vi "PositionCalibration2.vi"() -> ()   [LabVIEW 2017]
uses:
  <vilib>/Analysis/baseanly.llb/Mean (DBL).vi
  <vilib>/Instr/_visa.llb/VISA Configure Serial Port (Instr).vi
  <vilib>/Analysis/NI_AALBase.lvlib
panel:
  out "Digitial Signal":dbl
  out "Read Buffer":string
  out "Write Buffer":string
  in  "Sample Rate (Hz)":dbl
  in  "Baud Rate":i32(ring) items=["9600"=9600, "115200"=115200]
  in  "COM Port":refnum<visa-resource-name>
  in  "Stop":bool
  in  "Start":bool
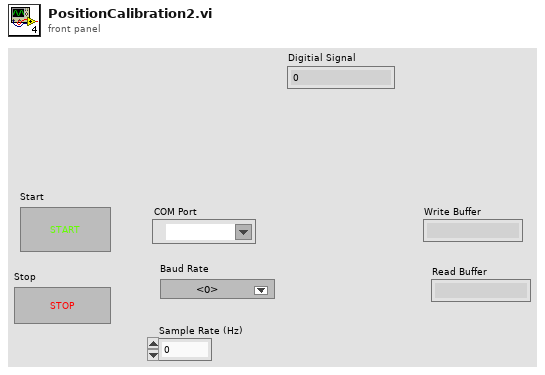
[diagram p1: front panel]
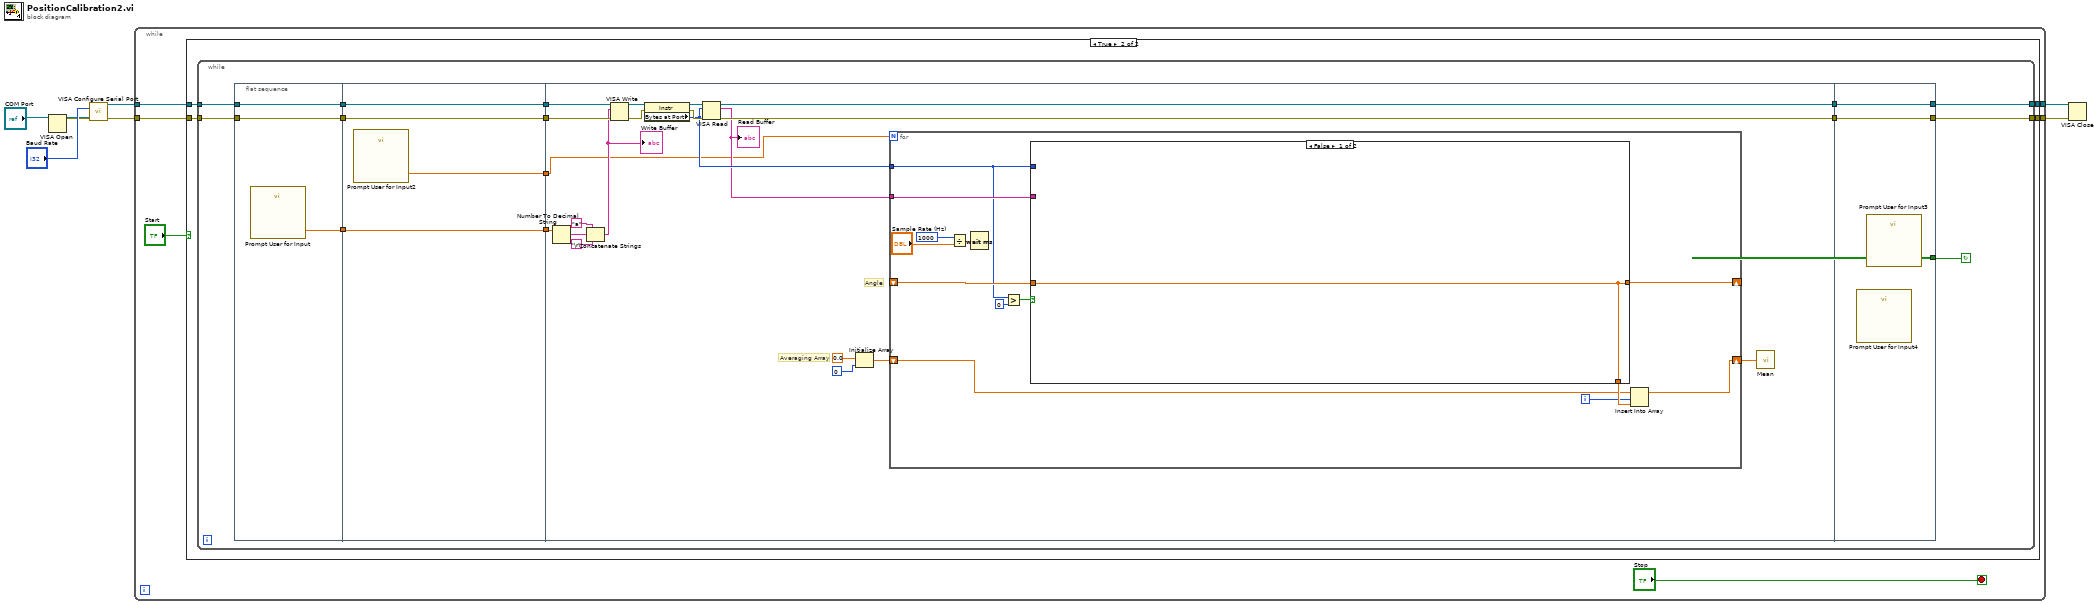
[diagram p0: block diagram]
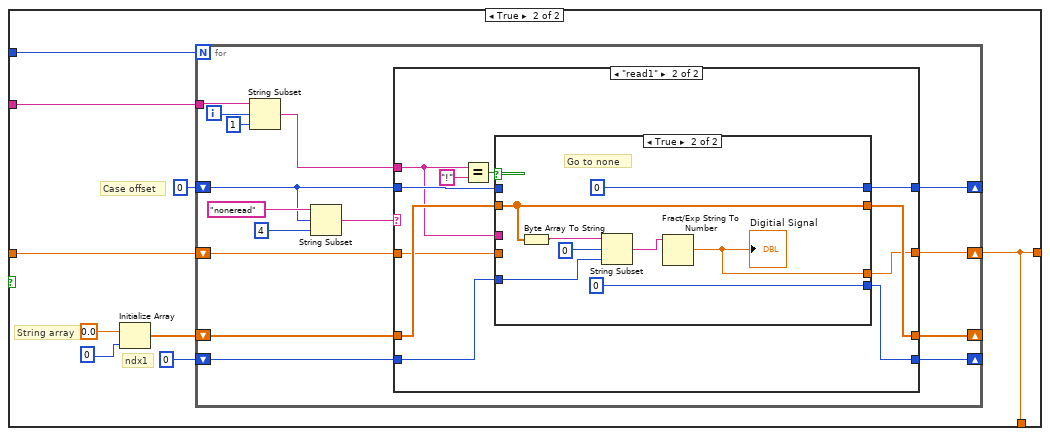
[diagram p3: hidden frame]
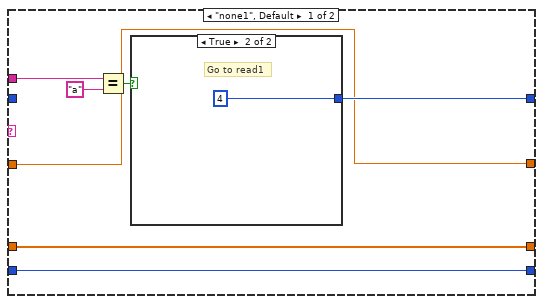
[diagram p4: hidden frame]
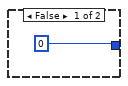
[diagram p5: hidden frame]
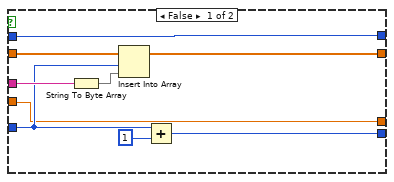
[diagram p6: hidden frame]
diagram:
  n1 = VISA Open(VISA resource name="COM Port") -> (VISA resource name=w6:refnum<visa-resource-name>, error out=w7:errorcluster)  [unwired: 4 in]
  n2 = call-poly "VISA Configure Serial Port"("VISA resource name"=w6, "baud rate (9600)"="Baud Rate", "error in (no error)"=w7) -> ("VISA resource name out"=w4:refnum<visa-resource-name>, "error out"=w3:errorcluster)  [unwired: 11 in]
  n3 = while {
    tunnel: w4 -> [w12]
    tunnel: w3 -> [w11]
    tunnel: [w10] -> w2
    tunnel: [w9] -> w1
    stop <- "Stop" stop-if-true
    n4 = case shown="True" "Start" {
      tunnel: w12 -> [w16 w20]
      tunnel: w11 -> [w15 w19]
      tunnel: [w16 w18] -> w10
      tunnel: [w15 w17] -> w9
      frame False {
      }
      frame True {
        n5 = while {
          tunnel: w20 -> [w30]
          tunnel: w19 -> [w26]
          tunnel: [w24] -> w18
          tunnel: [w22] -> w17
          stop <- w21 continue-if-true
          n6 = flat-sequence {
            tunnel: [w37] -> w34
            tunnel: [w36] -> w31
            tunnel: w30 -> [w36]
            tunnel: [w35] -> w27
            tunnel: w26 -> [w35]
            tunnel: w34 -> [w41]
            tunnel: [w41] -> w33
            tunnel: [w40] -> w32
            tunnel: w31 -> [w40]
            tunnel: [w39] -> w29
            tunnel: [w38] -> w28
            tunnel: w27 -> [w38]
            tunnel: w33 -> [w60]
            tunnel: w32 -> [w53]
            tunnel: w29 -> [w46]
            tunnel: w28 -> [w52]
            tunnel: [w50] -> w25
            tunnel: [w49] -> w23
            tunnel: w25 -> [w139]
            tunnel: [w139] -> w24
            tunnel: w23 -> [w138]
            tunnel: [w138] -> w22
            tunnel: [w137] -> w21
            frame #0 {
              n7 = call "Prompt User for Input"() -> ("Pwm"=w37:dbl)  [unwired: 17 in, 2 out]
            }
            frame #1 {
              n8 = call "Prompt User for Input2"() -> ("Number of Trials"=w39:dbl)  [unwired: 17 in, 2 out]
            }
            frame #2 {
              # "Averaging Array"
              # "Angle"
              n9 = Number To Decimal String(number=w60) -> (decimal integer string=w61:string)  [unwired: 1 in]
              n10 = Concatenate Strings("a", w61, "\r") -> (w51:string)
              "Write Buffer" <- w51
              n11 = VISA Write(VISA resource name=w53, write buffer=w51, error in (no error)=w52) -> (VISA resource name out=w57:refnum<visa-resource-name>, error out=w54:errorcluster)  [unwired: 1 out]
              n12 = property class="Instr"(reference=w57, error in=w54) -> (reference out=w56:refnum<visa-resource-name>, error out=w55:errorcluster, "Bytes at Port"=w48:u32)
              n13 = VISA Read(VISA resource name=w56, byte count=w48, error in (no error)=w55) -> (VISA resource name out=w50:refnum<visa-resource-name>, read buffer=w47:string, error out=w49:errorcluster)  [unwired: 1 out]
              "Read Buffer" <- w47
              n14 = Initialize Array(0.0 ("element"), 0 ("dimension size")) -> (w43:dbl[])
              n15 = for {
                N: w46 -> [_]
                tunnel: w48 -> [w69]
                tunnel: w47 -> [w74]
                shift-right: [w73] -> _
                shift-left: _ -> [w72]
                shift-right: [w63] -> w42
                shift-left: w43 -> [w64]
                i -> [w62]
                n16 = Divide(x=1000, y="Sample Rate (Hz)") -> (x/y=w68:dbl)
                n17 = Wait (ms)(milliseconds to wait=w68) -> ()  [unwired: 1 out]
                n18 = Greater?(x=w69, y=0) -> (0:w71:bool)
                n19 = case shown="False" w71 {
                  tunnel: w69 -> [_ w78]
                  tunnel: w74 -> [_ w84]
                  tunnel: [w75 w76] -> w65
                  tunnel: w72 -> [w75 w77]
                  tunnel: [w75 w76] -> w73
                  frame False {
                  }
                  frame True {
                    # "String array"
                    # "ndx1"
                    # "Case offset"
                    n20 = Initialize Array(0.0 ("element"), 0 ("dimension size")) -> (w79:dbl[])
                    n21 = for {
                      N: w78 -> [_]
                      tunnel: w84 -> [w98]
                      shift-right: [w94] -> _
                      shift-left: 0 -> [w88]
                      shift-right: [w93] -> _
                      shift-left: 0 -> [w92]
                      shift-right: [w90] -> _
                      shift-left: w79 -> [w91]
                      shift-right: [w85] -> w76
                      shift-left: w77 -> [w86]
                      i -> [w87]
                      n22 = String Subset(string=w98, offset (0)=w87, length (rest)=1 ("length (rest)")) -> (substring=w95:string)
                      n23 = String Subset(string="noneread", offset (0)=w88, length (rest)=4 ("length (rest)")) -> (substring=w89:string)
                      n24 = case shown="\"read1\"" w89 {
                        tunnel: w95 -> [w106 w109]
                        tunnel: [w103 w116] -> w94
                        tunnel: [w102 w112] -> w93
                        tunnel: w92 -> [w102 w113]
                        tunnel: w91 -> [w100 w114]
                        tunnel: [w100 w117] -> w90
                        tunnel: w88 -> [_ w115]
                        tunnel: [w101 w111] -> w85
                        tunnel: w86 -> [w101 w110]
                        frame "none1", Default {
                          n25 = Equal?(x=w106, y="a") -> (x = y?=w104:bool)
                          n26 = case shown="True" w104 {
                            tunnel: [0 4] -> w103
                            frame False {
                            }
                            frame True {
                              # "Go to read1"
                            }
                          }
                        }
                        frame "read1" {
                          n27 = Equal?(x=w109, y="!") -> (x = y?=w118:bool)
                          n28 = case shown="True" w118 {
                            tunnel: [w128 0] -> w112
                            tunnel: w114 -> [w122 w132]
                            tunnel: [w126 w132] -> w117
                            tunnel: w109 -> [w125 _]
                            tunnel: [w123 0] -> w116
                            tunnel: w115 -> [w123 _]
                            tunnel: w113 -> [w121 w131]
                            tunnel: [w120 w129] -> w111
                            tunnel: w110 -> [w120 _]
                            frame False {
                              n29 = String To Byte Array(string=w125) -> (unsigned byte array=w124:u8[])
                              n30 = Insert Into Array(array=w122, index=w121, new element=w124) -> (w126:dbl[])
                              n31 = Add(x=w121, y=1) -> (x+y=w128:i32)
                            }
                            frame True {
                              # "Go to none"
                              n32 = Byte Array To String(unsigned byte array=w132) -> (string=w133:string)
                              n33 = String Subset(string=w133, offset (0)=0, length (rest)=w131) -> (substring=w130:string)
                              n34 = Fract/Exp String To Number(string=w130) -> (number=w129:dbl)  [unwired: 3 in, 1 out]
                              "Digitial Signal" <- w129
                            }
                          }
                        }
                      }
                    }
                  }
                }
                n35 = Insert Into Array(array=w64, index=w62, new element=w65) -> (w63:dbl[])
              }
              n36 = call-poly <vilib>:"Mean.vi"("X"=w42) -> ()  [unwired: 2 out]
            }
            frame #3 {
              n37 = call "Prompt User for Input4"() -> ()  [unwired: 17 in, 3 out]
              n38 = call "Prompt User for Input3"() -> ("OK"=w137:bool)  [unwired: 18 in, 1 out]
            }
          }
        }
      }
    }
  }
  n39 = VISA Close(VISA resource name=w2, error in (no error)=w1) -> ()  [unwired: 1 out]
